vi "InitializeMotors.vi"() -> (0 "error out":errorcluster, 3 "WPI Robot":T1={"DevStatus"={"status"=FALSE, "code"=0, "source"=""}, "Motors[]"=[], "Square Inputs"=FALSE, "Max Output"=1.0})   [LabVIEW 2018]
uses:
  <vilib>/Rock Robotics/WPI/RobotDrive/WPI_RobotDriveDevRef.ctl
  <vilib>/Rock Robotics/WPI/MotorControl/WPI_MotorControlDeviceRef.ctl
  <vilib>/Rock Robotics/WPI/MotorControl/WPI_MotorControlType.ctl
  <vilib>/Rock Robotics/SystemInterfaces/DIO/FPGA_DIOPWMChannel.ctl
  <vilib>/Rock Robotics/WPI/PWM/WPI_PWMDeadband.ctl
  <vilib>/Rock Robotics/SystemInterfaces/DIO/FPGA_DIOChannel.ctl
  <vilib>/Rock Robotics/WPI/SafetyOutput/WPI_SafetyOutputConfigMenu.ctl
  <vilib>/Rock Robotics/WPI/ThirdParty/REV Robotics/SPARK MAX/Typedef/Spark MAX Motor Type.ctl
  <vilib>/Rock Robotics/WPI/RobotDrive/WPI_RobotDriveOpen2MotorWithExistingMotors.vi
panel:
  in  "PIDf Constants":cluster{"output max":dbl, "output min":dbl}={"output max"=1.0, "output min"=-1.0}
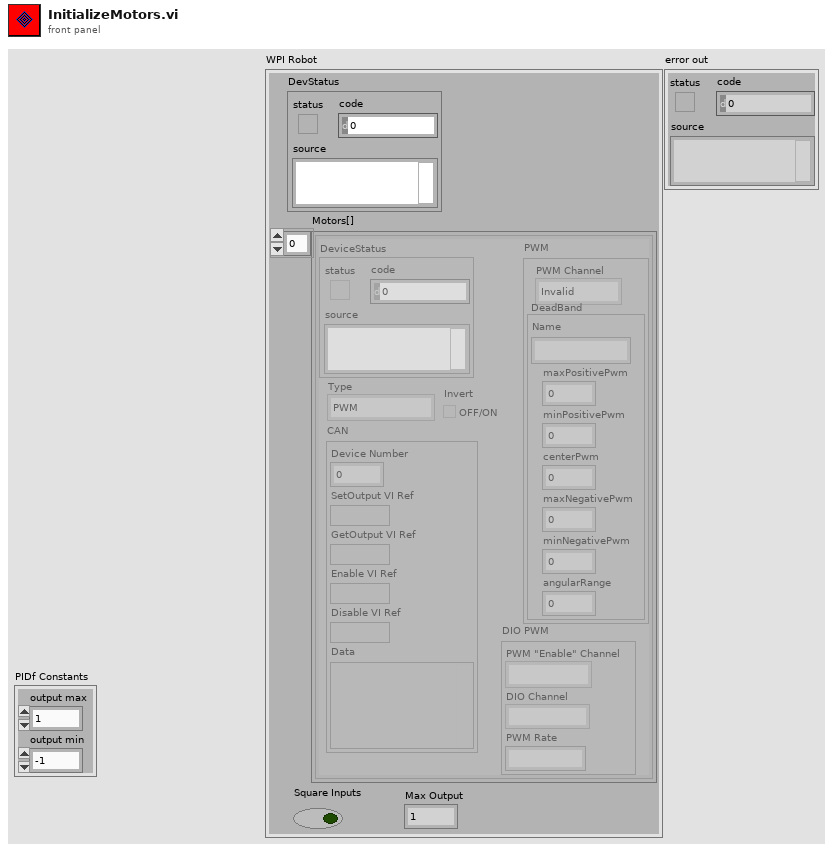
[diagram p1: front panel]
types:
  T1 = typedef "WPI_RobotDriveDevRef.ctl" = cluster{"DevStatus":errorcluster, "Motors[]":T2[], "Square Inputs":bool, "Max Output":dbl}
  T2 = typedef "WPI_MotorControlDeviceRef.ctl" = cluster{"DeviceStatus":errorcluster, "Type":T3, "PWM":cluster{"PWM Channel":T4, "DeadBand":T5}, "CAN":cluster{"Device Number":u8, "SetOutput VI Ref":variant, "GetOutput VI Ref":variant, "Enable VI Ref":variant, "Disable VI Ref":variant, "Data":variant}, "Invert":bool, "DIO PWM":cluster{"PWM \"Enable\" Channel":T4, "DIOChannel":T6, "PWM Rate":dbl}}
  T3 = typedef "WPI_MotorControlType.ctl" = enum16{"PWM", "CAN", "DIO PWM"}
  T4 = typedef "FPGA_DIOPWMChannel.ctl" = enum8{"PWM 0", "PWM 1", "PWM 2", "PWM 3", "PWM 4", "PWM 5", "PWM 6", "PWM 7", "PWM 8", "PWM 9", "PWM MXP 0", "PWM MXP 1", "PWM MXP 2", "PWM MXP 3", "PWM MXP 4", "PWM MXP 5", "PWM MXP 6", "PWM MXP 7", "PWM MXP 8", "PWM MXP 9", "Invalid"}
  T5 = typedef "WPI_PWMDeadband.ctl" = cluster{"Name":string, "maxPositivePwm":i32, "minPositivePwm":i32, "centerPwm":i32, "maxNegativePwm":i32, "minNegativePwm":i32, "angularRange":u16}
  T6 = typedef "FPGA_DIOChannel.ctl" = enum8{"DIO 0", "DIO 1", "DIO 2", "DIO 3", "DIO 4", "DIO 5", "DIO 6", "DIO 7", "DIO 8", "DIO 9", "DIO MXP 0", "DIO MXP 1", "DIO MXP 2", "DIO MXP 3", "DIO MXP 4", "DIO MXP 5", "DIO MXP 6", "DIO MXP 7", "DIO MXP 8", "DIO MXP 9", "DIO MXP 10", "DIO MXP 11", "DIO MXP 12", "DIO MXP 13", "DIO MXP 14", "DIO MXP 15", "SPI Port CS1", "SPI Port CS2", "SPI Port CS3", "SPI Port MISO", "SPI Port MOSI", "Invalid"}
  T7 = typedef "Spark MAX Motor Type.ctl" = enum16{"Brushed", "Brushless"}
  T8 = typedef "WPI_SafetyOutputConfigMenu.ctl" = enum16{"Enable", "Disable"}
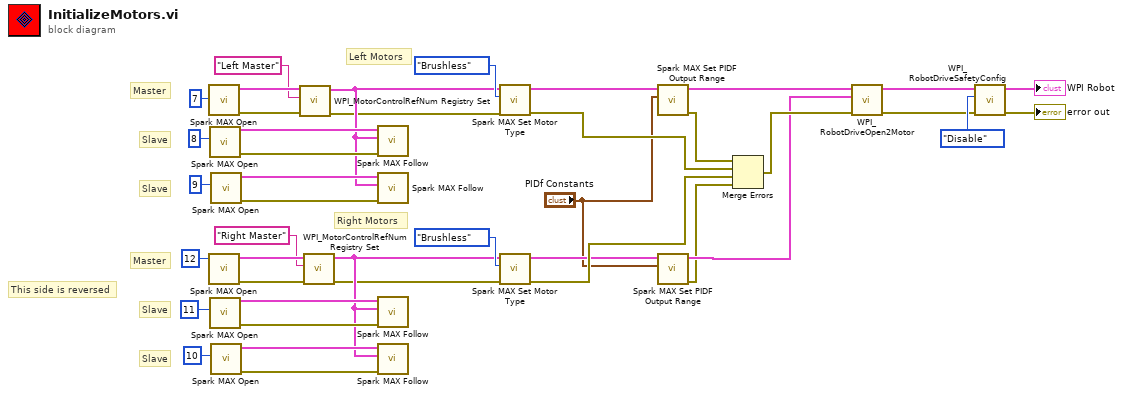
[diagram p0: block diagram]
diagram:
  # "This side is reversed"
  # "Slave"
  # "Slave"
  # "Master"
  # "Slave"
  # "Slave"
  # "Master"
  # "Right Motors"
  # "Left Motors"
  n1 = call <vilib>:"Spark MAX Open.vi"("Device Number"=u8 7) -> ("error out"=w15:errorcluster, "MotorControlDeviceRef"=w17:T2)  [unwired: 9 in]
  n2 = call <vilib>:"Spark MAX Open.vi"("Device Number"=u8 12) -> ("error out"=w10:errorcluster, "MotorControlDeviceRef"=w12:T2)  [unwired: 9 in]
  n3 = call <vilib>:"Spark MAX Open.vi"("Device Number"=u8 8) -> ("error out"=w41:errorcluster, "MotorControlDeviceRef"=w38:T2)  [unwired: 9 in]
  n4 = call <vilib>:"Spark MAX Open.vi"("Device Number"=u8 11) -> ("error out"=w29:errorcluster, "MotorControlDeviceRef"=w32:T2)  [unwired: 9 in]
  n5 = call <vilib>:"Spark MAX Open.vi"("Device Number"=u8 9) -> ("error out"=w36:errorcluster, "MotorControlDeviceRef"=w37:T2)  [unwired: 9 in]
  n6 = call <vilib>:"Spark MAX Open.vi"("Device Number"=u8 10) -> ("error out"=w23:errorcluster, "MotorControlDeviceRef"=w33:T2)  [unwired: 9 in]
  n7 = call <vilib>:"WPI_MotorControlRefNum Registry Set.vi"("error in (no error)"=w15, "refnum name"="Left Master", "MotorControlDevRef"=w17) -> ("error out"=w14:errorcluster, "MotorControlDevRef"=w16:T2)  [unwired: 7 in]
  n8 = call <vilib>:"WPI_MotorControlRefNum Registry Set.vi"("error in (no error)"=w10, "refnum name"="Right Master", "MotorControlDevRef"=w12) -> ("error out"=w9:errorcluster, "MotorControlDevRef"=w11:T2)  [unwired: 7 in]
  n9 = call <vilib>:"Spark MAX Follow.vi"("error in (no error)"=w41, "Master Controller"=w16, "MotorControlDeviceRef"=w38) -> ()  [unwired: 7 in, 2 out]
  n10 = call <vilib>:"Spark MAX Follow.vi"("error in (no error)"=w36, "Master Controller"=w16, "MotorControlDeviceRef"=w37) -> ()  [unwired: 7 in, 2 out]
  n11 = call <vilib>:"Spark MAX Follow.vi"("error in (no error)"=w29, "Master Controller"=w11, "MotorControlDeviceRef"=w32) -> ()  [unwired: 7 in, 2 out]
  n12 = call <vilib>:"Spark MAX Follow.vi"("error in (no error)"=w23, "Master Controller"=w11, "MotorControlDeviceRef"=w33) -> ()  [unwired: 7 in, 2 out]
  n13 = call <vilib>:"Spark MAX Set Motor Type.vi"("error in (no error)"=w14, "Enum"=Spark_MAX_Motor_Type."Brushless", "MotorControlDevRef"=w16) -> ("error out"=w22:errorcluster, "MotorControlDeviceRef"=w7:T2)  [unwired: 7 in]
  n14 = call <vilib>:"Spark MAX Set Motor Type.vi"("error in (no error)"=w9, "Enum"=Spark_MAX_Motor_Type."Brushless", "MotorControlDevRef"=w11) -> ("error out"=w21:errorcluster, "MotorControlDeviceRef"=w4:T2)  [unwired: 7 in]
  n15 = call <vilib>:"Spark MAX Set PIDF Output Range.vi"("output range"="PIDf Constants", "MotorControlDeviceRef"=w7) -> ("error out"=w1:errorcluster, "MotorControlDeviceRef"=w6:T2)  [unwired: 8 in]
  n16 = call <vilib>:"Spark MAX Set PIDF Output Range.vi"("output range"="PIDf Constants", "MotorControlDeviceRef"=w4) -> ("error out"=w2:errorcluster, "MotorControlDeviceRef"=w5:T2)  [unwired: 8 in]
  n17 = Merge Errors(w1, w22, w21, w2) -> (w20:errorcluster)
  n18 = call-poly <vilib>:"WPI_RobotDriveOpen2Motor.vi"("error in (no error)"=w20, "Right Motor Dev Ref"=w5, "Left Motor Dev Ref"=w6) -> ("error out"=w19:errorcluster, "RobotDriveDevRef"=w28:T1)  [unwired: 7 in]
  n19 = call <vilib>:"WPI_RobotDriveSafetyConfig.vi"("error in (no error)"=w19, "mode"=WPI_SafetyOutputConfigMenu."Disable", "RobotDriveDevRef"=w28) -> ("error out"=→"error out":errorcluster, "RobotDriveDevRef"=→"WPI Robot":T1)  [unwired: 7 in]
